vi "ReadAngle.vi"(8 "error in (no error)":errorcluster, 11 "ConfigParams":T2) -> (0 "error out":errorcluster, 3 "Cluster":T1)   [LabVIEW 2024]
uses:
  Ctrls/GlobalConfigure.ctl
  Ctrls/AngleVerify.ctl
  Excel.lvlibp
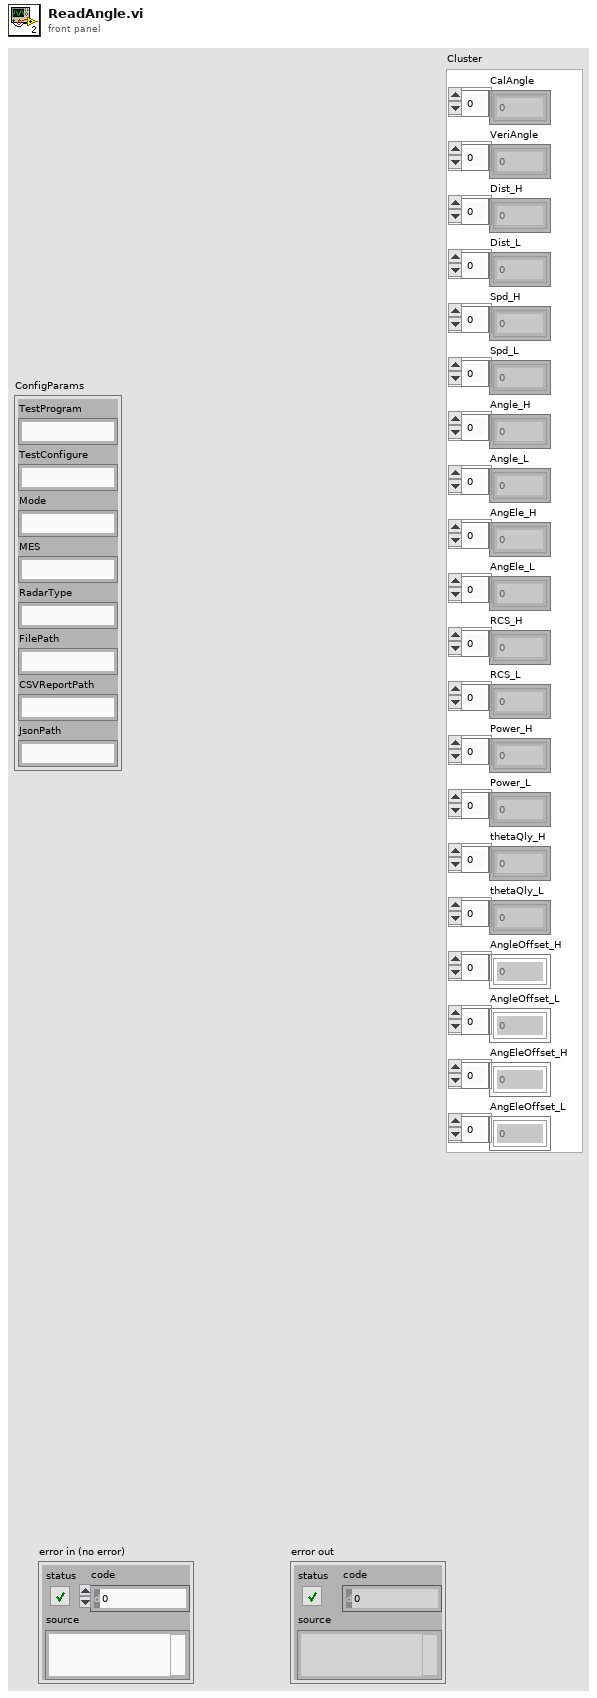
[diagram p1: front panel]
types:
  T1 = typedef "AngleVerify.ctl" = cluster{"CalAngle":dbl[], "VeriAngle":dbl[], "Dist_H":dbl[], "Dist_L":dbl[], "Spd_H":dbl[], "Spd_L":dbl[], "Angle_H":dbl[], "Angle_L":dbl[], "AngEle_H":dbl[], "AngEle_L":dbl[], "RCS_H":dbl[], "RCS_L":dbl[], "Power_H":dbl[], "Power_L":dbl[], "thetaQly_H":dbl[], "thetaQly_L":dbl[], "AngleOffset_H":dbl[], "AngleOffset_L":dbl[], "AngEleOffset_H":dbl[], "AngEleOffset_L":dbl[]}
  T2 = typedef "GlobalConfigure.ctl" = cluster{"TestProgram":string, "TestConfigure":string, "Mode":string, "MES":string, "RadarType":string, "FilePath":string, "CSVReportPath":string, "JsonPath":string}
  T3 = cluster{"Excel._Application":refnum<k7>, "Excel._Workbook":refnum<k7>, "Worksheets":refnum<k7>, "Excel._Worksheet":refnum<k7>, "Excel.Shapes":refnum<k7>, "Range":refnum<k7>}
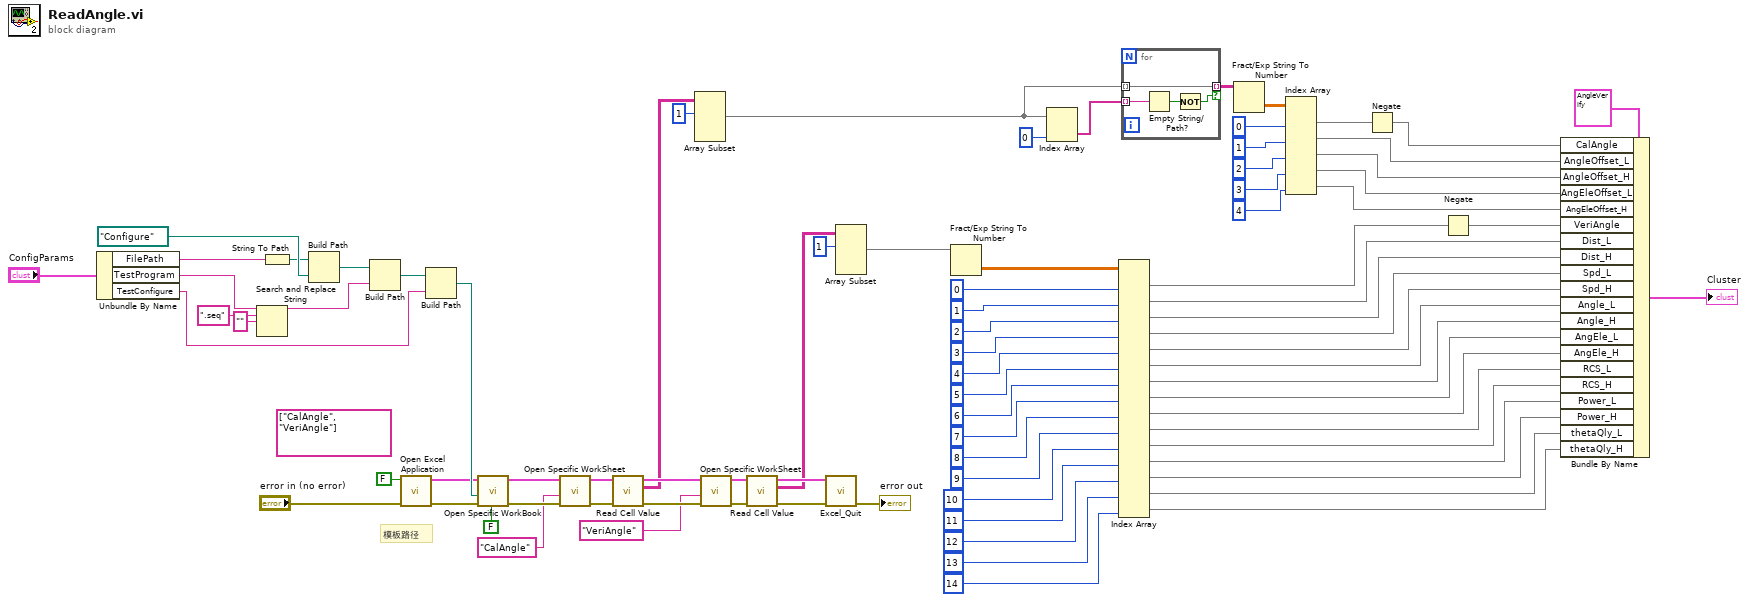
[diagram p0: block diagram]
diagram:
  (unwired) string[] ["CalAngle", "VeriAngle"]
  # "模板路径"
  n1 = Unbundle By Name("ConfigParams") -> ("FilePath"=w68:string, "TestProgram"=w72:string, "TestConfigure"=w77:string)
  n2 = Search and Replace String(input string=w72, search string=".seq" ("replace string (\"\")"), replace string="" ("replace string (\"\")")) -> (result string=w75:string)  [unwired: 5 in, 3 out]
  n3 = String To Path(string=w68) -> (path=w69:path)
  n4 = Build Path(base path=w69, name or relative path=path "Configure") -> (appended path=w71:path)
  n5 = Build Path(base path=w71, name or relative path=w75) -> (appended path=w76:path)
  n6 = call "Open Excel Application.vi"("error in (no error)"="error in (no error)", "Visible?"=FALSE) -> ("error out"=w81:errorcluster, "Excel Ref out"=w80:T3)  [unwired: 4 in]
  n7 = Build Path(base path=w76, name or relative path=w77) -> (appended path=w85:path)
  n8 = call "Open Specific WorkBook.vi"("Create"=FALSE, "error in (no error)"=w81, "path"=w85, "Excel Ref in"=w80) -> ("error out"=w79:errorcluster, "Excel Ref out"=w78:T3)  [unwired: 4 in]
  n9 = call "Open Specific WorkSheet.vi"("error in (no error)"=w79, "Name"="CalAngle", "Excel Ref in"=w78) -> ("error out"=w42:errorcluster, "Excel Ref out"=w43:T3)  [unwired: 2 in, 1 out]
  n10 = call "Read Cell Value.vi"("error in (no error)"=w42, "Excel Ref in"=w43) -> ("error out"=w37:errorcluster, "Value Array"=w15:string[][], "Excel Ref out"=w38:T3)  [unwired: 5 in]
  n11 = Array Subset(array=w15, index (row)=1 ("index")) -> (w14:string[][])  [unwired: 3 in]
  n12 = call "Open Specific WorkSheet.vi"("error in (no error)"=w37, "Name"="VeriAngle", "Excel Ref in"=w38) -> ("error out"=w40:errorcluster, "Excel Ref out"=w39:T3)  [unwired: 2 in, 1 out]
  n13 = call "Read Cell Value.vi"("error in (no error)"=w40, "Excel Ref in"=w39) -> ("error out"=w35:errorcluster, "Value Array"=w33:string[][], "Excel Ref out"=w34:T3)  [unwired: 5 in]
  n14 = call "Excel_Quit.vi"("Excel Ref in"=w34, "error in"=w35) -> ("error out"=→"error out":errorcluster)  [unwired: 13 in]
  n15 = Array Subset(array=w33, index (row)=1 ("index")) -> (w63:string[][])  [unwired: 3 in]
  n16 = Fract/Exp String To Number(string=w63) -> (number=w62:dbl[][])  [unwired: 3 in, 1 out]
  n17 = Index Array(array=w14, index (col)=0 ("disabled index (col)")) -> (element=w31:string[])  [unwired: 1 in]
  n18 = Index Array(array=w62, index (col) #1=0 ("disabled index (col)"), index (col) #2=1 ("disabled index (col)"), index (col) #3=2 ("disabled index (col)"), index (col) #4=3 ("disabled index (col)"), index (col) #5=4 ("disabled index (col)"), index (col) #6=5 ("disabled index (col)"), index (col) #7=6 ("disabled index (col)"), index (col) #8=7 ("disabled index (col)"), index (col) #9=8 ("disabled index (col)"), index (col) #10=9 ("disabled index (col)"), index (col) #11=10 ("disabled index (col)"), index (col) #12=11 ("disabled index (col)"), index (col) #13=12 ("disabled index (col)"), index (col) #14=13 ("disabled index (col)"), index (col) #15=14 ("disabled index (col)")) -> (element #1=w52:dbl[], element #2=w51:dbl[], element #3=w50:dbl[], element #4=w49:dbl[], element #5=w48:dbl[], element #6=w47:dbl[], element #7=w46:dbl[], element #8=w45:dbl[], element #9=w44:dbl[], element #10=w22:dbl[], element #11=w21:dbl[], element #12=w20:dbl[], element #13=w19:dbl[], element #14=w18:dbl[], element #15=w17:dbl[])  [unwired: 15 in]
  n19 = for {
    tunnel: w31 -> [w89] mode=indexing
    tunnel: [w86] -> w13 mode=indexing if=w87
    tunnel: w14 -> [w86] mode=indexing
    n20 = Empty String/Path?(string/path=w89) -> (empty?=w88:bool)
    n21 = Not(x=w88) -> (.not. x?=w87:bool)
  }
  n22 = Fract/Exp String To Number(string=w13) -> (number=w7:dbl[][])  [unwired: 3 in, 1 out]
  n23 = Index Array(array=w7, index (col) #1=0 ("disabled index (col)"), index (col) #2=1 ("disabled index (col)"), index (col) #3=2 ("disabled index (col)"), index (col) #4=3 ("disabled index (col)"), index (col) #5=4 ("disabled index (col)")) -> (element #1=w6:dbl[], element #2=w4:dbl[], element #3=w3:dbl[], element #4=w2:dbl[], element #5=w1:dbl[])  [unwired: 5 in]
  n24 = Negate(x=w6) -> (-x=w5:dbl[])
  n25 = Negate(x=w52) -> (-x=w32:dbl[])
  n26 = Bundle By Name(cluster=T1 {"CalAngle"=[], "VeriAngle"=[], "Dist_H"=[], "Dist_L"=[], "Spd_H"=[], "Spd_L"=[], "Angle_H"=[], "Angle_L"=[], "AngEle_H"=[], "AngEle_L"=[], "RCS_H"=[], "RCS_L"=[], "Power_H"=[], "Power_L"=[], "thetaQly_H"=[], "thetaQly_L"=[], "AngleOffset_H"=[], "AngleOffset_L"=[], "AngEleOffset_H"=[], "AngEleOffset_L"=[]} ("Cluster"), "CalAngle"=w5, "AngleOffset_L"=w4, "AngleOffset_H"=w3, "AngEleOffset_L"=w2, "AngEleOffset_H"=w1, "VeriAngle"=w32, "Dist_L"=w51, "Dist_H"=w50, "Spd_L"=w49, "Spd_H"=w48, "Angle_L"=w47, "Angle_H"=w46, "AngEle_L"=w45, "AngEle_H"=w44, "RCS_L"=w22, "RCS_H"=w21, "Power_L"=w20, "Power_H"=w19, "thetaQly_L"=w18, "thetaQly_H"=w17) -> (→"Cluster":T1)
